vi "Send Log String Data.vi"(0 "Message Enqueuer":refnum<class "Message Enqueuer.lvclass">, 1 "Message Priority (Normal)":T1=enum."Normal", 5 "Group Name (Untitled)":string, 7 "Channel Names (Untitled)":string[](array[string]), 9 "Data":string[][](array[string]), 11 "error in (no error)":errorcluster) -> (4 "Message Enqueuer out":refnum<class "Message Enqueuer.lvclass">, 15 "error out":errorcluster)   [LabVIEW 2024, in "Data Logger Actor Interface.lvlib" / "Log String Data Msg.lvclass"]
doc: "This VI sends the message to an actor."
uses:
  Log String Data Msg.lvclass
  <vilib>/ActorFramework/Message Enqueuer/Message Enqueuer.lvclass
  <vilib>/ActorFramework/Message Enqueuer/Message Priority.ctl
  C:/Program Files (x86)/National Instruments/LabVIEW 2024/vi.lib/ActorFramework/Message/Message.lvclass
  Log String Data Msg.lvclass/Log String Data Msg.ctl
  <vilib>/ActorFramework/Message Enqueuer/Message Enqueuer.lvclass/Message Enqueuer.ctl
  <vilib>/ActorFramework/Message Priority Queue/Priority Enqueue.vi
  C:/Users/uspoaotto/OneDrive - Oregon Tool/Desktop/working copies/dataLogger/Data Logger Actor Interface/Data Logger Actor Interface Messages/Log String Data Msg/Log String Data Msg.lvclass
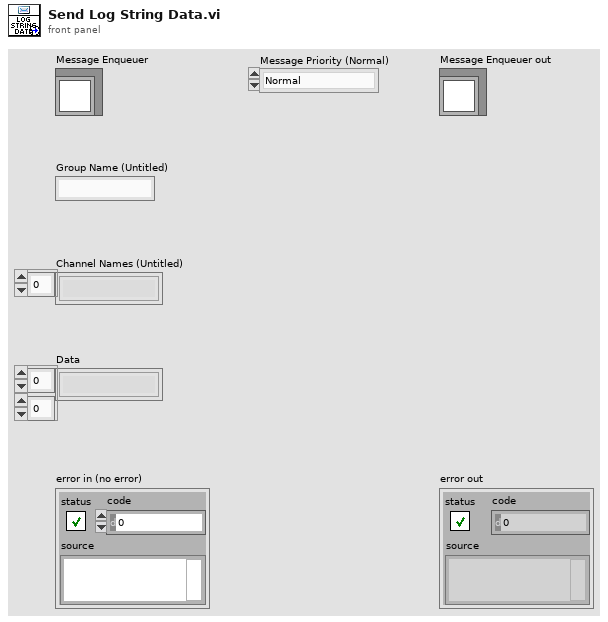
[diagram p1: front panel]
types:
  T1 = typedef "Actor Framework.lvlib/Message Enqueuer.lvclass/Message Priority.ctl" = enum16{"Low", "Normal", "High"}
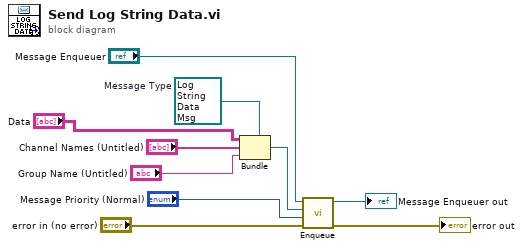
[diagram p0: block diagram]
diagram:
  w4 = refnum<class "Log String Data Msg.lvclass"> refnum  # Message Type
  n1 = Bundle(cluster=w4, "Data", "Channel Names (Untitled)", "Group Name (Untitled)") -> (w5:refnum<class "Log String Data Msg.lvclass">)
  n2 = call <vilib>:"Enqueue.vi"("error in (no error)"="error in (no error)", "Message Priority (Normal)"="Message Priority (Normal)", "Message"=w5, "Message Enqueuer in"="Message Enqueuer") -> ("error out"=→"error out":errorcluster, "Message Enqueuer out"=→"Message Enqueuer out":refnum<class "Message Enqueuer.lvclass">)  [unwired: 6 in]
